vi "server hello world.vi"() -> ()   [LabVIEW 2016]
uses:
  server/lvlibretls server listener.lvclass
  C:/Users/IEUser/Desktop/tlssimple/libretls/context parent/lvlibretls configurable context.lvclass
  context parent/lvlibretls configurable context.lvclass
  socket connection/lvlibretls connection.lvclass
panel:
  out "error out":errorcluster
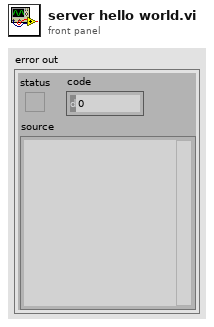
[diagram p1: front panel]
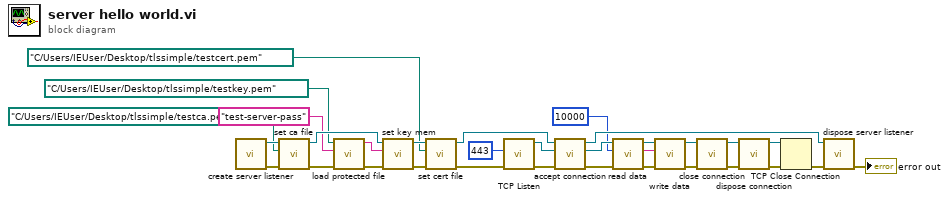
[diagram p0: block diagram]
diagram:
  n1 = call "create server listener.vi"() -> ("error out"=w31:errorcluster, "lvlibretls server listener out"=w32:refnum<class "lvlibretls server listener.lvclass">)  [unwired: 10 in]
  n2 = call "set ca file.vi"("error in"=w31, "ca file"=path "C:/Users/IEUser/Desktop/tlssimple/testca.pem", "lvlibretls configurable context in"=w32) -> ("error out"=w7:errorcluster, "lvlibretls configurable context out"=w6:refnum<class "lvlibretls server listener.lvclass">)  [unwired: 7 in]
  n3 = call "load protected file.vi"("error in"=w7, "password"="test-server-pass", "Path"=path "C:/Users/IEUser/Desktop/tlssimple/testkey.pem" ("key file")) -> ("error out"=w10:errorcluster, "data"=w11:string)  [unwired: 7 in]
  n4 = call "set key mem.vi"("error in"=w10, "key file"=w11, "lvlibretls configurable context in"=w6) -> ("error out"=w8:errorcluster, "lvlibretls configurable context out"=w9:refnum<class "lvlibretls server listener.lvclass">)  [unwired: 7 in]
  n5 = call "set cert file.vi"("error in"=w8, "cert file"=path "C:/Users/IEUser/Desktop/tlssimple/testcert.pem" ("ca file"), "lvlibretls configurable context in"=w9) -> ("error out"=w4:errorcluster, "lvlibretls configurable context out"=w5:refnum<class "lvlibretls server listener.lvclass">)  [unwired: 7 in]
  n6 = call <vilib>:"TCP Listen.vi"("error in (no error)"=w4, "port"=u16 443) -> ("error out"=w27:errorcluster, "connection ID"=w28:refnum<k5>)  [unwired: 5 in, 3 out]
  n7 = call "accept connection.vi"("error in"=w27, "connection ID"=w28, "lvlibretls server listener in"=w5) -> ("error out"=w19:errorcluster, "lvlibretls connection"=w20:refnum<class "lvlibretls connection.lvclass">, "lvlibretls server listener out"=w21:refnum<class "lvlibretls server listener.lvclass">)  [unwired: 6 in]
  n8 = call "read data.vi"("error in"=w19, "max size"=10000, "lvlibretls connection in"=w20) -> ("error out"=w17:errorcluster, "data"=w14:string, "lvlibretls connection out"=w18:refnum<class "lvlibretls connection.lvclass">)  [unwired: 6 in]
  n9 = call "write data.vi"("error in"=w17, "data"=w14, "lvlibretls connection in"=w18) -> ("error out"=w15:errorcluster, "lvlibretls connection out"=w16:refnum<class "lvlibretls connection.lvclass">)  [unwired: 7 in]
  n10 = call "close connection.vi"("error in"=w15, "lvlibretls connection in"=w16) -> ("error out"=w25:errorcluster, "lvlibretls connection out"=w26:refnum<class "lvlibretls connection.lvclass">)  [unwired: 8 in]
  n11 = call "dispose connection.vi"("error in"=w25, "lvlibretls connection in"=w26) -> ("error out"=w24:errorcluster, "connection"=w22:refnum<k5>)  [unwired: 8 in]
  n12 = TCP Close Connection(connection ID=w22, error in (no error)=w24) -> (error out=w23:errorcluster)  [unwired: 1 in, 1 out]
  n13 = call "dispose server listener.vi"("error in"=w23, "lvlibretls server listener in"=w21) -> ("error out"=→"error out":errorcluster)  [unwired: 9 in]
